vi "Logging - Usr Ev Class properties Template.vi"() -> ()   [LabVIEW 2023, in "Logging.lvlib" / "Logging_Class.lvclass"]
uses:
  Logging_Class.lvclass
  Logging - Ctrl - Usr Ev Ref.ctl
  Logging - Ctrl - Usr Ev Reg - Refs.ctl
  <vilib>/ActorFramework/Message Enqueuer/Message Enqueuer.lvclass
panel:
  out "Class Cluster Template":T3
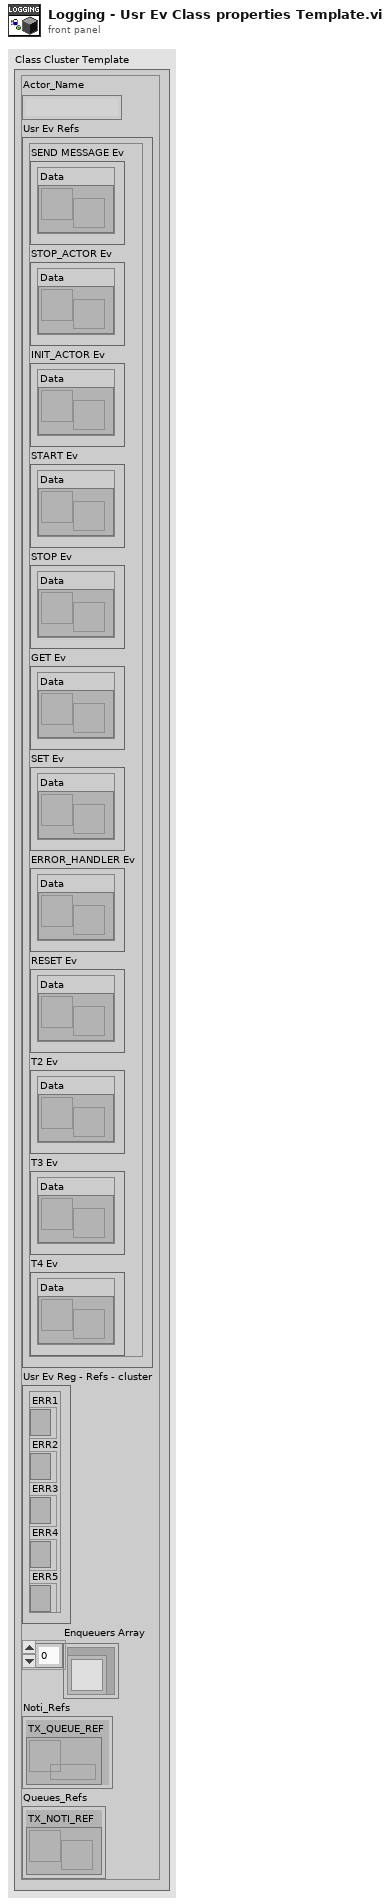
[diagram p1: front panel]
types:
  T1 = typedef "Logging.lvlib/Logging_Class.lvclass/Logging - Ctrl - Usr Ev Ref.ctl" = cluster{"SEND MESSAGE Ev":cluster{"Data":refnum<user-event>}, "STOP_ACTOR Ev":cluster{"Data":refnum<user-event>}, "INIT_ACTOR Ev":cluster{"Data":refnum<user-event>}, "START Ev":cluster{"Data":refnum<user-event>}, "STOP Ev":cluster{"Data":refnum<user-event>}, "GET Ev":cluster{"Data":refnum<user-event>}, "SET Ev":cluster{"Data":refnum<user-event>}, "ERROR_HANDLER Ev":cluster{"Data":refnum<user-event>}, "RESET Ev":cluster{"Data":refnum<user-event>}, "T2 Ev":cluster{"Data":refnum<user-event>}, "T3 Ev":cluster{"Data":refnum<user-event>}, "T4 Ev":cluster{"Data":refnum<user-event>}}
  T2 = typedef "Logging.lvlib/Logging_Class.lvclass/Logging - Ctrl - Usr Ev Reg - Refs.ctl" = cluster{"ERR1":refnum<event-registration>, "ERR2":refnum<event-registration>, "ERR3":refnum<event-registration>, "ERR4":refnum<event-registration>, "ERR5":refnum<event-registration>}
  T3 = cluster{"Actor_Name":string, "Usr Ev Refs":T1, "Usr Ev Reg - Refs - cluster":T2, "Enqueuers Array":refnum<class "Message Enqueuer.lvclass">[], "Noti_Refs":cluster{"TX_QUEUE_REF":refnum<queue>}, "Queues_Refs":cluster{"TX_NOTI_REF":refnum<notifier>}}
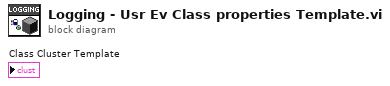
[diagram p0: block diagram]
diagram:
